vi "testUpload_raw2.vi"() -> ()   [LabVIEW 2025]
panel:
  out "error out 3":errorcluster
  out "error out 2":errorcluster
  out "Device":i32
  out "device 2":enum16{"CPU", "GPU0"}(ring)=enum."GPU0"
  in  "device":enum16{"CPU", "GPU0"}(ring)=enum."GPU0"
  out "loadedImgSucc":i32
  out "error out":errorcluster
  in  "PathImage":path=path "D:/Test/dllTest/images_2"
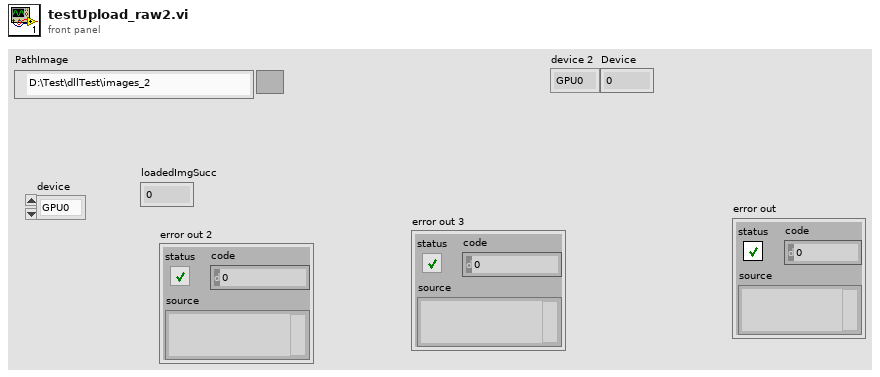
[diagram p1: front panel]
types:
  T1 = typedef "IMAQ Image.ctl" = refnum<image>
  T2 = enum32{"Map Pixel Pointer", "Unmap Pixel Pointer", "Get Pixels Infos"}
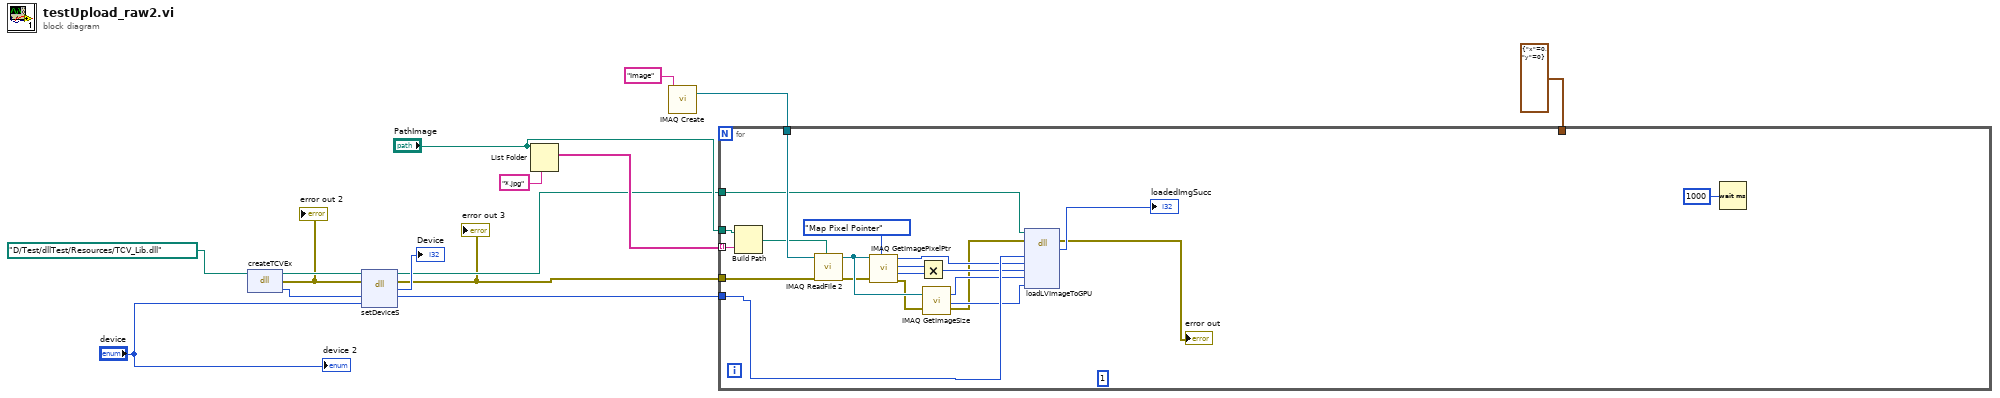
[diagram p0: block diagram]
diagram:
  n1 = dll-call lib="D:/Test/adslvPackageDev/Resources/TCV_Lib.dll" fn="createTCVEx"(path in=path "D:/Test/dllTest/Resources/TCV_Lib.dll") -> (path out=w8:path, error out=w2:errorcluster, "tcv"=w7:u64)  [unwired: 2 in]
  "error out 2" <- w2
  n2 = dll-call lib="D:/Test/dllTest/Resources/TCV_Lib.dll" fn="setDeviceS"(path in=w8, error in=w2, "tcv"=w7, "device"="device") -> (path out=w3:path, error out=w1:errorcluster, "Device"=→"Device":i32, "tcv"=w6:u64)  [unwired: 2 in]
  "error out 3" <- w1
  n3 = List Folder(path="PathImage", pattern="*.jpg") -> (filenames=w11:string[])  [unwired: 2 in, 3 out]
  n4 = call "IMAQ Create"("Image Name"="Image") -> ("New Image"=w14:T1)  [unwired: 4 in, 1 out]
  n5 = for {
    tunnel: "PathImage" -> [w36]
    tunnel: w14 -> [w33]
    tunnel: cluster{"x":i32, "y":i32} {"x"=0, "y"=0} -> [_]
    tunnel: w11 -> [w34] mode=indexing
    tunnel: w6 -> [w26]
    tunnel: w3 -> [w27]
    tunnel: w1 -> [w18]
    (unwired) 1 ("norm")
    n6 = Build Path(base path=w36, name or relative path=w34) -> (appended path=w32:path)
    n7 = call "IMAQ ReadFile 2"("File Path"=w32, "error in (no error)"=w18, "Image"=w33) -> ("error out"=w17:errorcluster, "Image Out"=w28:T1)  [unwired: 4 in, 3 out]
    n8 = call "IMAQ GetImagePixelPtr"("Function"=T2."Map Pixel Pointer", "error in (no error)"=w17, "Image"=w28) -> ("error out"=w16:errorcluster, "Pixel Size (Bytes)"=w30:i32, "LineWidth(Pixels)"=w29:i32, "Pixel Pointer out"=w25:u64)  [unwired: 3 in, 2 out]
    n9 = Multiply(x=w29, y=w30) -> (x*y=w24:i32)
    n10 = call "IMAQ GetImageSize"("Image"=w28, "error in (no error)"=w16) -> ("Y Resolution"=w23:i32, "X Resolution"=w22:i32, "error out"=w19:errorcluster)  [unwired: 2 in]
    n11 = dll-call lib="D:/Test/dllTest/Resources/TCV_Lib.dll" fn="loadLVImageToGPU"(path in=w27, error in=w19, "tcv"=w26, "lvImgPtr"=w25, "lw"=w24, "h"=w23, "w"=w22) -> (error out=→"error out":errorcluster, "succ"=→"loadedImgSucc":i32)  [unwired: 6 in, 1 out]
    n12 = Wait (ms)(milliseconds to wait=u32 1000) -> ()  [unwired: 1 out]
  }
  "device 2" <- "device"
